vi "Get Configuration Version.vi"() -> (3 "Version":T1={"Major"=1, "Minor"=0, "Fix"=0, "Build"=0})   [LabVIEW 2020, in "ADAS PE Template.lvlib" / "ADAS PE Template.lvclass"]
doc: "<b>Get Configuration Version</b>\nSpecify the current serialized configuration version of the <b>Configuration.ctl</b> typedef. This is used to mutate previously serialized configurations to the current format if changes are made."
uses:
  ADAS PE Template.lvclass
  <vilib>/ADAS Record/Utilities/TypeDefs/Config Version.ctl
  <vilib>/ADAS Record/Utilities/ADAS Utilities.lvlib
panel:
  # "Specify the current serialized configuration version of the Configuration.ctl typedef. This is used to mutate previously serialized configurations to the current format if changes are made."
  # "#via_ignore"
  # "**Update on Block Diagram**"
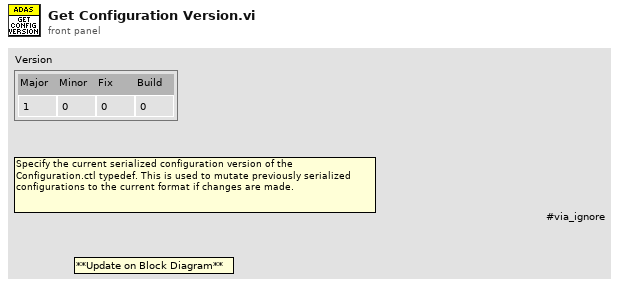
[diagram p1: front panel]
types:
  T1 = typedef "ADAS Utilities.lvlib/Config Version.ctl" = cluster{"Major":u32, "Minor":u32, "Fix":u32, "Build":u32}
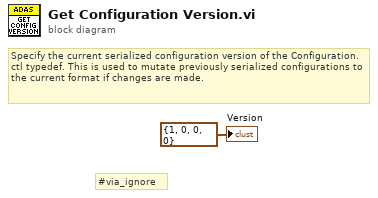
[diagram p0: block diagram]
diagram:
  # "#via_ignore"
  # "Specify the current serialized configuration version of the Configuration.ctl typedef. This is used to mutate previously serialized configurations to the current format if changes are made."
  "Version" <- T1 {"Major"=1, "Minor"=0, "Fix"=0, "Build"=0} ("Version")
